vi "update_frd_data.vi"(11 "experiment-data":T1) -> (3 "FrdData Out":T3)   [LabVIEW 2017]
uses:
  controls/FrdData.ctl
  controls/SS_FourierData.ctl
  controls/SS_experimental-data.ctl
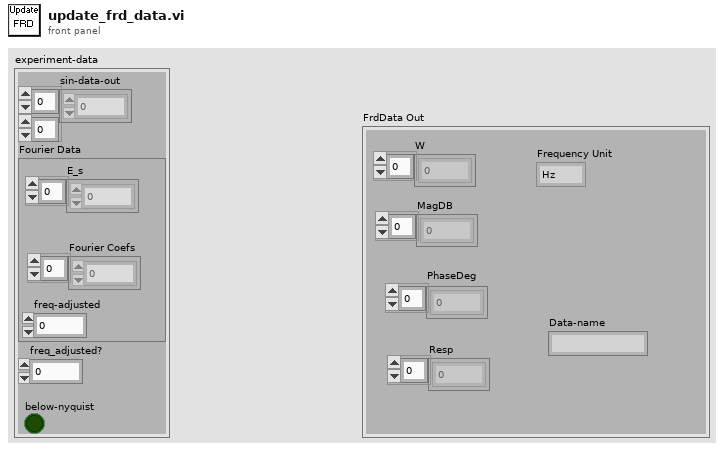
[diagram p1: front panel]
types:
  T1 = typedef "SS_experimental-data.ctl" = cluster{"sin-data-out":dbl[][], "Fourier Data":T2, "freq_adjusted?":dbl, "below-nyquist":bool}
  T2 = typedef "SS_FourierData.ctl" = cluster{"E_s":dbl[], "Fourier Coefs":cdb[], "freq-adjusted":dbl}
  T3 = typedef "FrdData.ctl" = cluster{"Frequency Unit":enum16{"Hz", "rad/s"}, "W":dbl[], "MagDB":dbl[], "PhaseDeg":dbl[], "Resp":cdb[], "Data-name":string}
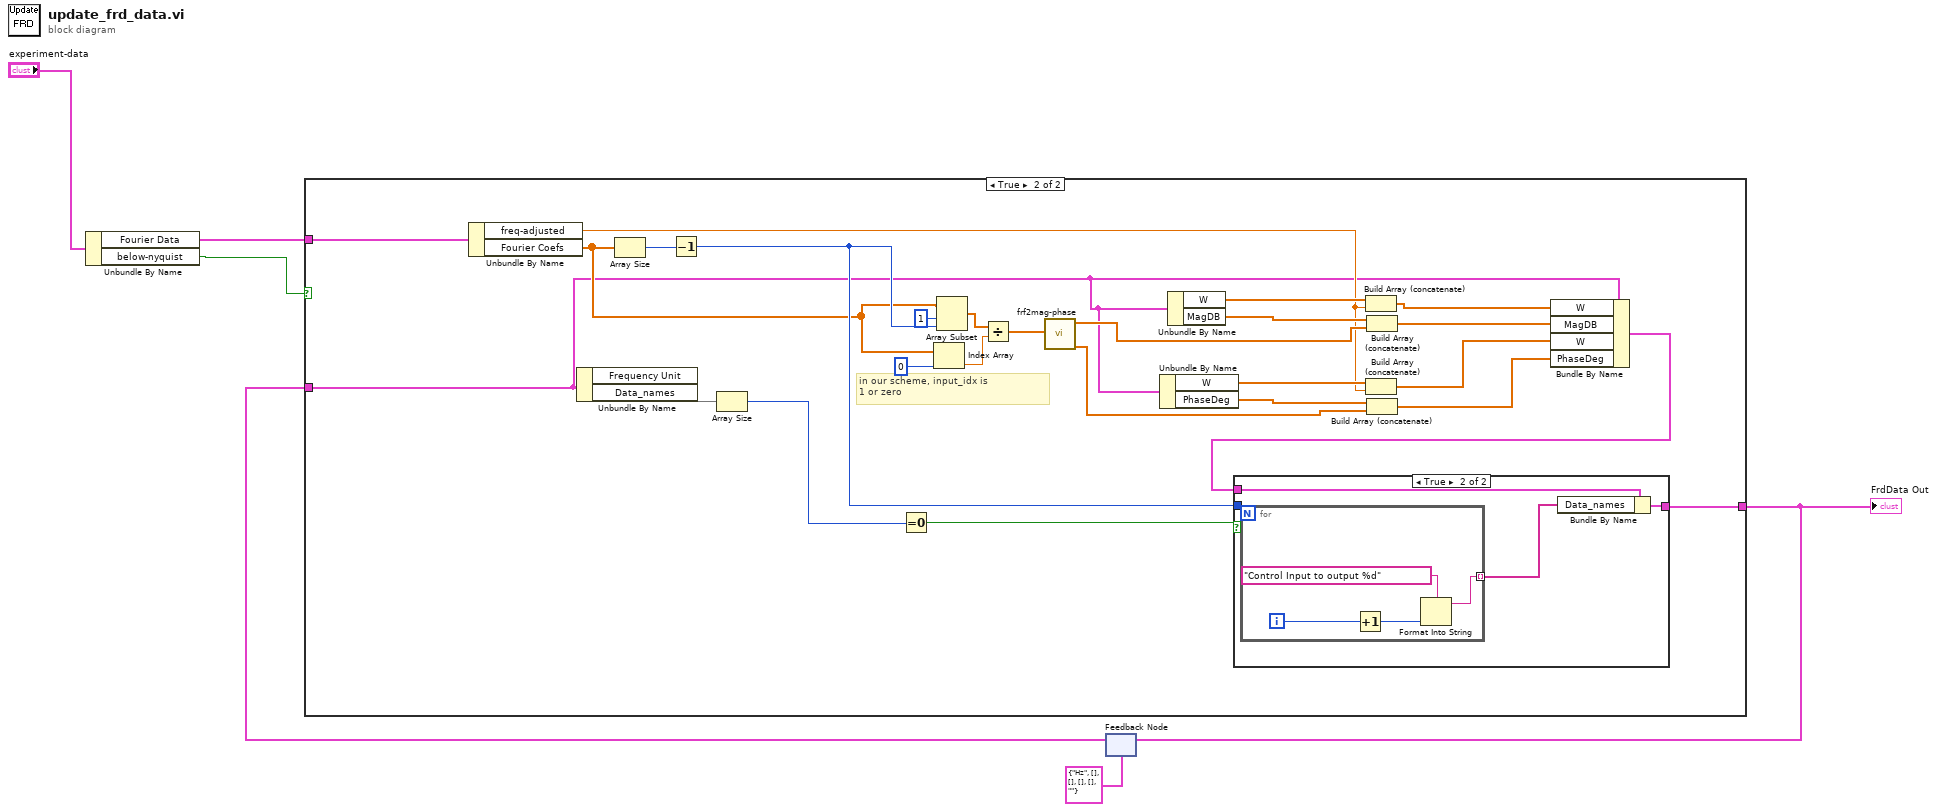
[diagram p0: block diagram]
diagram:
  n1 = Unbundle By Name("experiment-data") -> ("Fourier Data"=w4:T2, "below-nyquist"=w1:bool)
  n2 = feedback #1(T3 {"Frequency Unit"=enum."Hz", "W"=[], "MagDB"=[], "PhaseDeg"=[], "Resp"=[], "Data-name"=""} ("FrdData Out 2")) -> (w3:T3)
  n3 = case shown="True" w1 {
    tunnel: [w7 w13] -> w6
    tunnel: w4 -> [_ w9]
    tunnel: w3 -> [w7 w8]
    frame False {
    }
    frame True {
      # "in our scheme, input_idx is\n1 or zero"
      n4 = Unbundle By Name(w9) -> ("freq-adjusted"=w10:dbl, "Fourier Coefs"=w11:cdb[])
      n5 = Unbundle By Name(w8) -> ("Data_names"=w33)  [unwired: 1 out]
      n6 = Array Size(array=w11) -> (size(s)=w32:i32)
      n7 = Decrement(x=w32) -> (x-1=w15:i32)
      n8 = Array Size(array=w33) -> (size(s)=w31:i32)
      n9 = Equal To 0?(x=w31) -> (x = 0?=w30:bool)
      n10 = Index Array(array=w11, index=0) -> (element=w29:cdb)
      n11 = Array Subset(array=w11, index=1, length=w15) -> (w25:cdb[])
      n12 = Divide(x=w25, y=w29) -> (x/y=w24:cdb[])
      n13 = call "frf2mag-phase.vi"("G_frf"=w24) -> ("phase [deg]"=w12:dbl[], "mag-dB"=w28:dbl[])  [unwired: 9 in]
      n14 = Unbundle By Name(w8) -> ("W"=w19:dbl[], "PhaseDeg"=w18:dbl[])
      n15 = Unbundle By Name(w8) -> ("W"=w23:dbl[], "MagDB"=w22:dbl[])
      n16 = Build Array (concatenate)(w23, w10) -> (w21:dbl[])
      n17 = Build Array (concatenate)(w19, w10) -> (w17:dbl[])
      n18 = Build Array (concatenate)(w22, w28) -> (w20:dbl[])
      n19 = Build Array (concatenate)(w18, w12) -> (w16:dbl[])
      n20 = Bundle By Name(cluster=w8, "W"=w21, "MagDB"=w20, "W"=w17, "PhaseDeg"=w16) -> (w14:T3)
      n21 = case shown="True" w30 {
        tunnel: w15 -> [_ w38]
        tunnel: w14 -> [w34 w37]
        tunnel: [w34 w35] -> w13
        frame False {
        }
        frame True {
          n22 = for {
            N: w38 -> [_]
            tunnel: [w39] -> w36 mode=indexing
            i -> [w42]
            n23 = Increment(x=w42) -> (x+1=w41:i32)
            n24 = Format Into String(format string="Control Input to output %d", w41) -> (resulting string=w39:string)  [unwired: 2 in, 1 out]
          }
          n25 = Bundle By Name(cluster=w37, "Data_names"=w36) -> (w35:T3)
        }
      }
    }
  }
  "FrdData Out" <- w6
  n26 = feedback-in #1(w6) -> ()
